vi "Write Nesting level.vi"(8 "error in (no error)":errorcluster, 10 "Nesting level":i16, 11 "Element-XML in":refnum<class "Element-XML.lvclass">) -> (0 "error out":errorcluster, 3 "Element-XML out":refnum<class "Element-XML.lvclass">)   [LabVIEW 2013, in "HardwareCharacterization.lvlib" / "Element-XML.lvclass"]
uses:
  Element-XML.lvclass
  Element-XML.lvclass/Element-XML.ctl
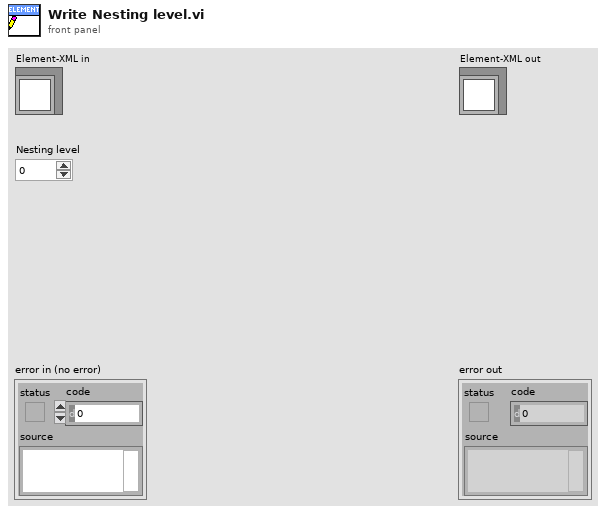
[diagram p1: front panel]
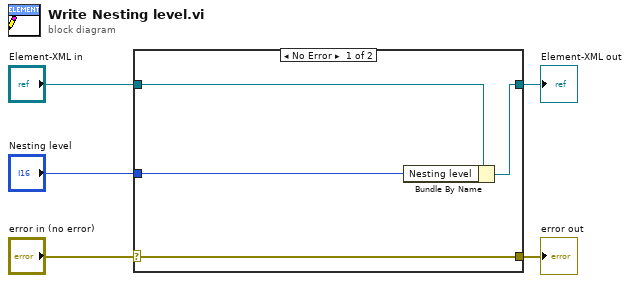
[diagram p0: block diagram]
diagram:
  n1 = case shown="No Error" "error in (no error)" {
    selector: "error in (no error)" -> [w9 w10]
    tunnel: [w9 w10] -> w4
    tunnel: [w7 w11] -> w2
    tunnel: "Element-XML in" -> [w8 w11]
    tunnel: "Nesting level" -> [w6 _]
    frame No Error {
      n2 = Bundle By Name(cluster=w8, "Nesting level"=w6) -> (w7:refnum<class "Element-XML.lvclass">)
    }
    frame Error {
    }
  }
  "error out" <- w4
  "Element-XML out" <- w2
